vi "Func-엑셀 데이터를 그래프로 출력.vi"() -> ()   [LabVIEW 2015] (continued)
29.418\n25\t25\t29.423\n25\t25\t29.426\n25\t25\t29.429\n25\t25\t29.431\n25\t25\t29.437\n25\t25\t29.438\n25\t25\t29.442\n25\t25\t29.448\n25\t25\t29.456\n25\t25\t29.462\n25\t25\t29.462\n25\t25\t29.467\n25\t25\t29.473\n25\t25\t29.48\n25\t25\t29.483\n25\t25\t29.488\n25\t25\t29.499\n25\t25\t29.505\n25\t25\t29.508\n25\t25\t29.516\n25\t25\t29.517\n25\t25\t29.518\n25\t25\t29.519\n25\t25\t29.522\n25\t25\t29.527\n25\t25\t29.529\n25\t25\t29.536\n25\t25\t29.544\n25\t25\t29.548\n25\t25\t29.554\n25\t25\t29.559\n25\t25\t29.562\n25\t25\t29.565\n25\t25\t29.569\n25\t25\t29.576\n25\t25\t29.58\n25\t25\t29.585\n25\t25\t29.589\n25\t25\t29.595\n25\t25\t29.598\n25\t25\t29.604\n25\t25\t29.607\n25\t25\t29.609\n25\t25\t29.611\n25\t25\t29.611\n25\t25\t29.617\n25\t25\t29.616\n25\t25\t29.621\n25\t25\t29.626\n25\t25\t29.632\n25\t25\t29.64\n25\t25\t29.644\n25\t25\t29.651\n25\t25\t29.655\n25\t25\t29.661\n25\t25\t29.664\n25\t25\t29.663\n25\t25\t29.668\n25\t25\t29.669\n25\t25\t29.671\n25\t25\t29.68\n25\t25\t29.681\n25\t25\t29.686\n25\t25\t29.693\n25\t25\t29.7\n25\t25\t29.705\n25\t25\t29.707\n25\t25\t29.713\n25\t25\t29.716\n25\t25\t29.72\n25\t25\t29.721\n25\t25\t29.728\n25\t25\t29.73\n25\t25\t29.73\n25\t25\t29.734\n25\t25\t29.736\n25\t25\t29.74\n25\t25\t29.743\n25\t25\t29.75\n25\t25\t29.755\n25\t25\t29.756\n25\t25\t29.76\n25\t25\t29.762\n25\t25\t29.768\n25\t25\t29.77\n25\t25\t29.772\n25\t25\t29.783\n25\t25\t29.79\n25\t25\t29.794\n25\t25\t29.8\n25\t25\t29.803\n25\t25\t29.809\n25\t25\t29.811\n25\t25\t29.811\n25\t25\t29.815\n25\t25\t29.818\n25\t25\t29.825\n25\t25\t29.829\n25\t25\t29.836\n25\t25\t29.842\n25\t25\t29.846\n25\t25\t29.851\n25\t25\t29.854\n25\t25\t29.855\n25\t25\t29.859\n25\t25\t29.861\n25\t25\t29.866\n25\t25\t29.871\n25\t25\t29.871\n25\t25\t29.877\n25\t25\t29.881\n25\t25\t29.884\n25\t25\t29.885\n25\t25\t29.889\n25\t25\t29.894\n25\t25\t29.899\n25\t25\t29.902\n25\t25\t29.906\n25\t25\t29.913\n25\t25\t29.916\n25\t25\t29.92\n25\t25\t29.92\n25\t25\t29.923\n25\t25\t29.926\n25\t25\t29.927\n25\t25\t29.932\n25\t25\t29.935\n25\t25\t29.942\n25\t25\t29.949\n25\t25\t29.954\n25\t25\t29.964\n25\t25\t29.962\n25\t25\t29.966\n25\t25\t29.97\n25\t25\t29.97\n25\t25\t29.972\n25\t25\t29.972\n25\t25\t29.977\n25\t25\t29.982\n25\t25\t29.986\n25\t25\t29.99\n25\t25\t29.996\n25\t25\t30.006\n25\t25\t30.008\n25\t25\t30.011\n25\t25\t30.013\n25\t25\t30.017\n25\t25\t30.014\n25\t25\t30.016\n25\t25\t30.017\n25\t25\t30.025\n25\t25\t30.032\n25\t25\t30.036\n25\t25\t30.043\n25\t25\t30.047\n25\t25\t30.054\n25\t25\t30.055\n25\t25\t30.056\n25\t25\t30.061\n25\t25\t30.066\n25\t25\t30.069\n25\t25\t30.07\n25\t25\t30.075\n25\t25\t30.079\n25\t25\t30.083\n25\t25\t30.087\n25\t25\t30.093\n25\t25\t30.096\n25\t25\t30.098\n25\t25\t30.1\n25\t25\t30.098\n25\t25\t30.101\n25\t25\t30.104\n25\t25\t30.11\n25\t25\t30.114\n25\t25\t30.115\n25\t25\t30.119\n25\t25\t30.125\n25\t25\t30.127\n25\t25\t30.129\n25\t25\t30.138\n25\t25\t30.145\n25\t25\t30.15\n25\t25\t30.153\n25\t25\t30.154\n25\t25\t30.158\n25\t25\t30.154\n25\t25\t30.16\n25\t25\t30.165\n25\t25\t30.168\n25\t25\t30.174\n25\t25\t30.18\n25\t25\t30.186\n25\t25\t30.186\n25\t25\t30.19\n25\t25\t30.194\n25\t25\t30.197\n25\t25\t30.2\n25\t25\t30.203\n25\t25\t30.207\n25\t25\t30.212\n25\t25\t30.214\n25\t25\t30.218\n25\t25\t30.225\n25\t25\t30.226\n25\t25\t30.229\n25\t25\t30.229\n25\t25\t30.233\n25\t25\t30.234\n25\t25\t30.236\n25\t25\t30.243\n25\t25\t30.245\n25\t25\t30.249\n25\t25\t30.251\n25\t25\t30.253\n25\t25\t30.257\n25\t25\t30.257\n25\t25\t30.259\n25\t25\t30.264\n25\t25\t30.267\n25\t25\t30.272\n25\t25\t30.276\n25\t25\t30.282\n25\t25\t30.29\n25\t25\t30.293\n25\t25\t30.297\n25\t25\t30.302\n25\t25\t30.301\n25\t25\t30.301\n25\t25\t30.305\n25\t25\t30.306\n25\t25\t30.307\n25\t25\t30.312\n25\t25\t30.32\n25\t25\t30.326\n25\t25\t30.333\n25\t25\t30.338\n25\t25\t30.342\n25\t25\t30.343\n25\t25\t30.341\n25\t25\t30.346\n25\t25\t30.348\n25\t25\t30.346\n25\t25\t30.347\n25\t25\t30.352\n25\t25\t30.359\n25\t25\t30.356\n25\t25\t30.36\n25\t25\t30.366\n25\t25\t30.37\n25\t25\t30.372\n25\t25\t30.371\n25\t25\t30.38\n25\t25\t30.378\n25\t25\t30.381\n25\t25\t30.389\n25\t25\t30.391\n25\t25\t30.395\n25\t25\t30.399\n25\t25\t30.407\n25\t25\t30.41\n25\t25\t30.412\n25\t25\t30.415\n25\t25\t30.418\n25\t25\t30.422\n25\t25\t30.425\n25\t25\t30.431\n25\t25\t30.43\n25\t25\t30.434\n25\t25\t30.438\n25\t25\t30.443\n25\t25\t30.443\n25\t25\t30.442\n25\t25\t30.45\n25\t25\t30.452\n25\t25\t30.455\n25\t25\t30.459\n25\t25\t30.465\n25\t25\t30.468\n25\t25\t30.47\n25\t25\t30.471\n25\t25\t30.475\n25\t25\t30.477\n25\t25\t30.478\n25\t25\t30.484\n25\t25\t30.491\n25\t25\t30.495\n25\t25\t30.495\n25\t25\t30.5\n25\t25\t30.5\n25\t25\t30.503\n25\t25\t30.504\n25\t25\t30.51\n25\t25\t30.514\n25\t25\t30.516\n25\t25\t30.524\n25\t25\t30.529\n25\t25\t30.531\n25\t25\t30.533\n25\t25\t30.537\n25\t25\t30.539\n25\t25\t30.54\n25\t25\t30.54\n25\t25\t30.546\n25\t25\t30.547\n25\t25\t30.55\n25\t25\t30.553\n25\t25\t30.555\n25\t25\t30.558\n25\t25\t30.558\n25\t25\t30.562\n25\t25\t30.564\n25\t25\t30.567\n25\t25\t30.571\n25\t25\t30.573\n25\t25\t30.58\n25\t25\t30.579\n25\t25\t30.582\n25\t25\t30.583\n25\t25\t30.587\n25\t25\t30.591\n25\t25\t30.588\n25\t25\t30.589\n25\t25\t30.592\n25\t25\t30.597\n25\t25\t30.598\n25\t25\t30.603\n25\t25\t30.608\n25\t25\t30.616\n25\t25\t30.625\n25\t25\t30.629\n25\t25\t30.63\n25\t25\t30.635\n25\t25\t30.638\n25\t25\t30.637\n25\t25\t30.637\n25\t25\t30.64\n25\t25\t30.645\n25\t25\t30.647\n25\t25\t30.651\n25\t25\t30.659\n25\t25\t30.663\n25\t25\t30.665\n25\t25\t30.668\n25\t25\t30.668\n25\t25\t30.67\n25\t25\t30.672\n25\t25\t30.673\n25\t25\t30.677\n25\t25\t30.681\n25\t25\t30.686\n25\t25\t30.688\n25\t25\t30.691\n25\t25\t30.696\n25\t25\t30.697\n25\t25\t30.702\n25\t25\t30.705\n25\t25\t30.704\n25\t25\t30.707\n25\t25\t30.707\n25\t25\t30.711\n25\t25\t30.715\n25\t25\t30.72\n25\t25\t30.723\n25\t25\t30.725\n25\t25\t30.73\n25\t25\t30.729\n25\t25\t30.73\n25\t25\t30.729\n25\t25\t30.739\n25\t25\t30.741\n25\t25\t30.739\n25\t25\t30.745\n25\t25\t30.748\n25\t25\t30.749\n25\t25\t30.749\n25\t25\t30.75\n25\t25\t30.756\n25\t25\t30.761\n25\t25\t30.763\n25\t25\t30.77\n25\t25\t30.771\n25\t25\t30.777\n25\t25\t30.779\n25\t25\t30.781\n25\t25\t30.782\n25\t25\t30.777\n25\t25\t30.783\n25\t25\t30.785\n25\t25\t30.784\n25\t25\t30.786\n25\t25\t30.79\n25\t25\t30.796\n25\t25\t30.799\n25\t25\t30.8\n25\t25\t30.802\n25\t25\t30.806\n25\t25\t30.806\n25\t25\t30.807\n25\t25\t30.809\n25\t25\t30.814\n25\t25\t30.818\n25\t25\t30.821\n25\t25\t30.827\n25\t25\t30.831\n25\t25\t30.837\n25\t25\t30.837\n25\t25\t30.841\n25\t25\t30.845\n25\t25\t30.846\n25\t25\t30.846\n25\t25\t30.848\n25\t25\t30.85\n25\t25\t30.854\n25\t25\t30.855\n25\t25\t30.856\n25\t25\t30.865\n25\t25\t30.864\n25\t25\t30.869\n25\t25\t30.87\n25\t25\t30.875\n25\t25\t30.88\n25\t25\t30.878\n25\t25\t30.88\n25\t25\t30.885\n25\t25\t30.888\n25\t25\t30.889\n25\t25\t30.892\n25\t25\t30.895\n25\t25\t30.9\n25\t25\t30.897\n25\t25\t30.901\n25\t25\t30.903\n25\t25\t30.901\n25\t25\t30.905\n25\t25\t30.908\n25\t25\t30.913\n25\t25\t30.914\n25\t25\t30.916\n25\t25\t30.921\n25\t25\t30.923\n25\t25\t30.922\n25\t25\t30.926\n25\t25\t30.93\n25\t25\t30.931\n25\t25\t30.937\n25\t25\t30.939\n25\t25\t30.947\n25\t25\t30.953\n25\t25\t30.956\n25\t25\t30.959\n25\t25\t30.961\n25\t25\t30.965\n25\t25\t30.965\n25\t25\t30.966\n25\t25\t30.968\n25\t25\t30.972\n25\t25\t30.975\n25\t25\t30.974\n25\t25\t30.975\n25\t25\t30.978\n25\t25\t30.981\n25\t25\t30.981\n25\t25\t30.98\n25\t25\t30.985\n25\t25\t30.988\n25\t25\t30.997\n25\t25\t30.998\n25\t25\t31.003\n25\t25\t31.009\n25\t25\t31.011\n25\t25\t31.013\n25\t25\t31.01\n25\t25\t31.012\n25\t25\t31.011\n25\t25\t31.014\n25\t25\t31.014\n25\t25\t31.019\n25\t25\t31.021\n25\t25\t31.026\n25\t25\t31.029\n25\t25\t31.029\n25\t25\t31.033\n25\t25\t31.03\n25\t25\t31.037\n25\t25\t31.038\n25\t25\t31.043\n25\t25\t31.048\n25\t25\t31.05\n25\t25\t31.054\n25\t25\t31.055\n25\t25\t31.054\n25\t25\t31.055\n25\t25\t31.05\n25\t25\t31.051\n25\t25\t31.054\n25\t25\t31.053\n25\t25\t31.059\n25\t25\t31.061\n25\t25\t31.066\n25\t25\t31.07\n25\t25\t31.073\n25\t25\t31.078\n25\t25\t31.08\n25\t25\t31.081\n25\t25\t31.083\n25\t25\t31.086\n25\t25\t31.084\n25\t25\t31.086\n25\t25\t31.084\n25\t25\t31.089\n25\t25\t31.093\n25\t25\t31.096\n25\t25\t31.103\n25\t25\t31.104\n25\t25\t31.108\n25\t25\t31.114\n25\t25\t31.115\n25\t25\t31.12\n25\t25\t31.12\n25\t25\t31.123\n25\t25\t31.126\n25\t25\t31.125\n25\t25\t31.129\n25\t25\t31.132\n25\t25\t31.134\n25\t25\t31.133\n25\t25\t31.139\n25\t25\t31.141\n25\t25\t31.144\n25\t25\t31.145\n25\t25\t31.146\n25\t25\t31.149\n25\t25\t31.149\n25\t25\t31.15\n25\t25\t31.148\n25\t25\t31.148\n25\t25\t31.148\n25\t25\t31.15\n25\t25\t31.154\n25\t25\t31.154\n25\t25\t31.159\n25\t25\t31.164\n25\t25\t31.168\n25\t25\t31.168\n25\t25\t31.171\n25\t25\t31.175\n25\t25\t31.179\n25\t25\t31.181\n25\t25\t31.185\n25\t25\t31.188\n25\t25\t31.19\n25\t25\t31.19\n25\t25\t31.186\n25\t25\t31.19\n25\t25\t31.192\n25\t25\t31.195\n25\t25\t31.196\n25\t25\t31.204\n25\t25\t31.208\n25\t25\t31.21\n25\t25\t31.213\n25\t25\t31.218\n25\t25\t31.219\n25\t25\t31.219\n25\t25\t31.225\n25\t25\t31.227\n25\t25\t31.228\n25\t25\t31.232\n25\t25\t31.237\n25\t25\t31.237\n25\t25\t31.234\n25\t25\t31.238\n25\t25\t31.241\n25\t25\t31.242\n25\t25\t31.241\n25\t25\t31.245\n25\t25\t31.252\n25\t25\t31.254\n25\t25\t31.255\n25\t25\t31.253\n25\t25\t31.256\n25\t25\t31.259\n25\t25\t31.26\n25\t25\t31.261\n25\t25\t31.263\n25\t25\t31.265\n25\t25\t31.265\n25\t25\t31.265\n25\t25\t31.266\n25\t25\t31.27\n25\t25\t31.274\n25\t25\t31.279\n25\t25\t31.284\n25\t25\t31.288\n25\t25\t31.29\n25\t25\t31.289\n25\t25\t31.288\n25\t25\t31.289\n25\t25\t31.289\n25\t25\t31.293\n25\t25\t31.297\n25\t25\t31.3\n25\t25\t31.303\n25\t25\t31.306\n25\t25\t31.309\n25\t25\t31.311\n25\t25\t31.312\n25\t25\t31.313\n25\t25\t31.319\n25\t25\t31.321\n25\t25\t31.32\n25\t25\t31.321\n25\t25\t31.323\n25\t25\t31.326\n25\t25\t31.328\n25\t25\t31.33\n25\t25\t31.334\n25\t25\t31.336\n25\t25\t31.335\n25\t25\t31.335\n25\t25\t31.334\n25\t25\t31.333\n25\t25\t31.338\n25\t25\t31.339\n25\t25\t31.346\n25\t25\t31.355\n25\t25\t31.359\n25\t25\t31.366\n25\t25\t31.37\n25\t25\t31.371\n25\t25\t31.37\n25\t25\t31.366\n25\t25\t31.368\n25\t25\t31.366\n25\t25\t31.365\n25\t25\t31.366\n25\t25\t31.368\n25\t25\t31.374\n25\t25\t31.378\n25\t25\t31.38\n25\t25\t31.383\n25\t25\t31.389\n25\t25\t31.396\n25\t25\t31.394\n25\t25\t31.393\n25\t25\t31.398\n25\t25\t31.398\n25\t25\t31.397\n25\t25\t31.391\n25\t25\t31.391\n25\t25\t31.393\n25\t25\t31.392\n25\t25\t31.396\n25\t25\t31.396\n25\t25\t31.405\n25\t25\t31.409\n25\t25\t31.412\n25\t25\t31.418\n25\t25\t31.42\n25\t25\t31.418\n25\t25\t31.422\n25\t25\t31.423\n25\t25\t31.423\n25\t25\t31.422\n25\t25\t31.423\n25\t25\t31.428\n25\t25\t31.426\n25\t25\t31.429\n25\t25\t31.429\n25\t25\t31.432\n25\t25\t31.432\n25\t25\t31.431\n25\t25\t31.436\n25\t25\t31.437\n25\t25\t31.441\n25\t25\t31.446\n25\t25\t31.449\n25\t25\t31.455\n25\t25\t31.458\n25\t25\t31.462\n25\t25\t31.462\n25\t25\t31.458\n25\t25\t31.457\n25\t25\t31.46\n25\t25\t31.462\n25\t25\t31.464\n25\t25\t31.467\n25\t25\t31.471\n25\t25\t31.477\n25\t25\t31.475\n25\t25\t31.474\n25\t25\t31.473\n25\t25\t31.477\n25\t25\t31.479\n25\t25\t31.478\n25\t25\t31.482\n25\t25\t31.486\n25\t25\t31.491\n25\t25\t31.496\n25\t25\t31.496\n25\t25\t31.5\n25\t25\t31.501\n25\t25\t31.503\n25\t25\t31.5\n25\t25\t31.499\n25\t25\t31.503\n25\t25\t31.504\n25\t25\t31.511\n25\t25\t31.512\n25\t25\t31.515\n25\t25\t31.517\n25\t25\t31.515\n25\t25\t31.516\n25\t25\t31.52\n25\t25\t31.517\n25\t25\t31.518\n25\t25\t31.52\n25\t25\t31.526\n25\t25\t31.525\n25\t25\t31.522\n25\t25\t31.528\n25\t25\t31.531\n25\t25\t31.533\n25\t25\t31.531\n25\t25\t31.532\n25\t25\t31.536\n25\t25\t31.534\n25\t25\t31.536\n25\t25\t31.534\n25\t25\t31.538\n25\t25\t31.546\n25\t25\t31.548\n25\t25\t31.547\n25\t25\t31.554\n25\t25\t31.561\n25\t25\t31.561\n25\t25\t31.565\n25\t25\t31.568\n25\t25\t31.573\n25\t25\t31.575\n25\t25\t31.575\n25\t25\t31.577\n25\t25\t31.573\n25\t25\t31.572\n25\t25\t31.575\n25\t25\t31.577\n25\t25\t31.577\n25\t25\t31.578\n25\t25\t31.583\n25\t25\t31.585\n25\t25\t31.587\n25\t25\t31.587\n25\t25\t31.592\n25\t25\t31.596\n25\t25\t31.596\n25\t25\t31.601\n25\t25\t31.604\n25\t25\t31.605\n25\t25\t31.608\n25\t25\t31.61\n25\t25\t31.611\n25\t25\t31.607\n25\t25\t31.607\n25\t25\t31.607\n25\t25\t31.602\n25\t25\t31.604\n25\t25\t31.607\n25\t25\t31.612\n25\t25\t31.612\n25\t25\t31.618\n25\t25\t31.621\n25\t25\t31.621\n25\t25\t31.62\n25\t25\t31.62\n25\t25\t31.625\n25\t25\t31.626\n25\t25\t31.626\n25\t25\t31.631\n25\t25\t31.637\n25\t25\t31.639\n25\t25\t31.641\n25\t25\t31.641\n25\t25\t31.65\n25\t25\t31.649\n25\t25\t31.65\n25\t25\t31.649\n25\t25\t31.652\n25\t25\t31.65\n25\t25\t31.651\n25\t25\t31.654\n25\t25\t31.656\n25\t25\t31.657\n25\t25\t31.655\n25\t25\t31.661\n25\t25\t31.659\n25\t25\t31.661\n25\t25\t31.661\n25\t25\t31.67\n25\t25\t31.674\n25\t25\t31.67\n25\t25\t31.671\n25\t25\t31.67\n25\t25\t31.668\n25\t25\t31.666\n25\t25\t31.664\n25\t25\t31.668\n25\t25\t31.671\n25\t25\t31.675\n25\t25\t31.68\n25\t25\t31.682\n25\t25\t31.686\n25\t25\t31.687\n25\t25\t31.69\n25\t25\t31.689\n25\t25\t31.691\n25\t25\t31.691\n25\t25\t31.693\n25\t25\t31.699\n25\t25\t31.698\n25\t25\t31.696\n25\t25\t31.698\n25\t25\t31.703\n25\t25\t31.702\n25\t25\t31.701\n25\t25\t31.704\n25\t25\t31.708\n25\t25\t31.707\n25\t25\t31.704\n25\t25\t31.71\n25\t25\t31.711\n25\t25\t31.714\n25\t25\t31.717\n25\t25\t31.72\n25\t25\t31.722\n25\t25\t31.721\n25\t25\t31.723\n25\t25\t31.723\n25\t25\t31.723\n25\t25\t31.727\n25\t25\t31.729\n25\t25\t31.733\n25\t25\t31.73\n25\t25\t31.735\n25\t25\t31.739\n25\t25\t31.736\n25\t25\t31.734\n25\t25\t31.735\n25\t25\t31.742\n25\t25\t31.743\n25\t25\t31.745\n25\t25\t31.75\n25\t25\t31.753\n25\t25\t31.755\n25\t25\t31.755\n25\t25\t31.757\n25\t25\t31.754\n25\t25\t31.755\n25\t25\t31.76\n25\t25\t31.763\n25\t25\t31.764\n25\t25\t31.764\n25\t25\t31.771\n25\t25\t31.77\n25\t25\t31.769\n25\t25\t31.771\n25\t25\t31.773\n25\t25\t31.774\n25\t25\t31.771\n25\t25\t31.777\n25\t25\t31.777\n25\t25\t31.779\n25\t25\t31.779\n25\t25\t31.781\n25\t25\t31.782\n25\t25\t31.779\n25\t25\t31.784\n25\t25\t31.787\n25\t25\t31.789\n25\t25\t31.791\n25\t25\t31.795\n25\t25\t31.798\n25\t25\t31.799\n25\t25\t31.801\n25\t25\t31.804\n25\t25\t31.804\n25\t25\t31.807\n25\t25\t31.811\n25\t25\t31.809\n25\t25\t31.81\n25\t25\t31.81\n25\t25\t31.811\n25\t25\t31.812\n25\t25\t31.813\n25\t25\t31.818\n25\t25\t31.821\n25\t25\t31.822\n25\t25\t31.823\n25\t25\t31.824\n25\t25\t31.823\n25\t25\t31.823\n25\t25\t31.821\n25\t25\t31.826\n25\t25\t31.826\n25\t25\t31.83\n25\t25\t31.832\n25\t25\t31.835\n25\t25\t31.838\n25\t25\t31.841\n25\t25\t31.847\n25\t25\t31.845\n25\t25\t31.845\n25\t25\t31.844\n25\t25\t31.844\n25\t25\t31.841\n25\t25\t31.841\n25\t25\t31.843\n25\t25\t31.844\n25\t25\t31.845\n25\t25\t31.848\n25\t25\t31.848\n25\t25\t31.849\n25\t25\t31.851\n25\t25\t31.854\n25\t25\t31.857\n25\t25\t31.855\n25\t25\t31.857\n25\t25\t31.861\n25\t25\t31.859\n25\t25\t31.862\n25\t25\t31.863\n25\t25\t31.864\n25\t25\t31.868\n25\t25\t31.869\n25\t25\t31.873\n25\t25\t31.874\n25\t25\t31.876\n25\t25\t31.878\n25\t25\t31.879\n25\t25\t31.882\n25\t25\t31.885\n25\t25\t31.883\n25\t25\t31.882\n25\t25\t31.882\n25\t25\t31.886\n25\t25\t31.885\n25\t25\t31.885\n25\t25\t31.888\n25\t25\t31.892\n25\t25\t31.895\n25\t25\t31.894\n25\t25\t31.895\n25\t25\t31.895\n25\t25\t31.898\n25\t25\t31.899\n25\t25\t31.901\n25\t25\t31.904\n25\t25\t31.906\n25\t25\t31.91\n25\t25\t31.911\n25\t25\t31.91\n25\t25\t31.909\n25\t25\t31.909\n25\t25\t31.909\n25\t25\t31.908\n25\t25\t31.911\n25\t25\t31.914\n25\t25\t31.917\n25\t25\t31.918\n25\t25\t31.921\n25\t25\t31.921\n25\t25\t31.922\n25\t25\t31.922\n25\t25\t31.925\n25\t25\t31.928\n25\t25\t31.927\n25\t25\t31.927\n25\t25\t31.928\n25\t25\t31.929\n25\t25\t31.927\n25\t25\t31.927\n25\t25\t31.93\n25\t25\t31.937\n25\t25\t31.936\n25\t25\t31.937\n25\t25\t31.942\n25\t25\t31.941\n25\t25\t31.941\n25\t25\t31.939\n25\t25\t31.942\n25\t25\t31.944\n25\t25\t31.947\n25\t25\t31.953\n25\t25\t31.955\n25\t25\t31.957\n25\t25\t31.96\n25\t25\t31.96\n25\t25\t31.961\n25\t25\t31.959\n25\t25\t31.958\n25\t25\t31.958\n25\t25\t31.957\n25\t25\t31.958\n25\t25\t31.959\n25\t25\t31.963\n25\t25\t31.966\n25\t25\t31.968\n25\t25\t31.968\n25\t25\t31.97\n25\t25\t31.973\n25\t25\t31.971\n25\t25\t31.976\n25\t25\t31.977\n25\t25\t31.979\n25\t25\t31.979\n25\t25\t31.978\n25\t25\t31.978\n25\t25\t31.976\n25\t25\t31.979\n25\t25\t31.981\n25\t25\t31.984\n25\t25\t31.987\n25\t25\t31.985\n25\t25\t31.989\n25\t25\t31.988\n25\t25\t31.992\n25\t25\t31.989\n25\t25\t31.989\n25\t25\t31.992\n25\t25\t31.991\n25\t25\t31.993\n25\t25\t31.993\n25\t25\t32\n25\t25\t32.006\n25\t25\t32.01\n25\t25\t32.011\n25\t25\t32.01\n25\t25\t32.012\n25\t25\t32.011\n25\t25\t32.008\n25\t25\t32.01\n25\t25\t32.011\n25\t25\t32.016\n25\t25\t32.016\n25\t25\t32.018\n25\t25\t32.021\n25\t25\t32.021\n25\t25\t32.022\n25\t25\t32.023\n25\t25\t32.024\n25\t25\t32.023\n25\t25\t32.021\n25\t25\t32.024\n25\t25\t32.023\n25\t25\t32.021\n25\t25\t32.022\n25\t25\t32.024\n25\t25\t32.027\n25\t25\t32.029\n25\t25\t32.03\n25\t25\t32.032\n25\t25\t32.036\n25\t25\t32.039\n25\t25\t32.038\n25\t25\t32.037\n25\t25\t32.042\n25\t25\t32.042\n25\t25\t32.043\n25\t25\t32.044\n25\t25\t32.047\n25\t25\t32.049\n25\t25\t32.048\n25\t25\t32.051\n25\t25\t32.051\n25\t25\t32.05\n25\t25\t32.048\n25\t25\t32.049\n25\t25\t32.048\n25\t25\t32.05\n25\t25\t32.056\n25\t25\t32.057\n25\t25\t32.061\n25\t25\t32.063\n25\t25\t32.066\n25\t25\t32.066\n25\t25\t32.064\n25\t25\t32.065\n25\t25\t32.066\n25\t25\t32.066\n25\t25\t32.067\n25\t25\t32.066\n25\t25\t32.069\n25\t25\t32.073\n25\t25\t32.071\n25\t25\t32.071\n25\t25\t32.072\n25\t25\t32.075\n25\t25\t32.074\n25\t25\t32.071\n25\t25\t32.078\n25\t25\t32.079\n25\t25\t32.078\n25\t25\t32.082\n25\t25\t32.083\n25\t25\t32.089\n25\t25\t32.086\n25\t25\t32.088\n25\t25\t32.091\n25\t25\t32.09\n25\t25\t32.09\n25\t25\t32.087\n25\t25\t32.087\n25\t25\t32.091\n25\t25\t32.095\n25\t25\t32.094\n25\t25\t32.095\n25\t25\t32.096\n25\t25\t32.099\n25\t25\t32.097\n25\t25\t32.093\n25\t25\t32.097\n25\t25\t32.104\n25\t25\t32.107\n25\t25\t32.108\n25\t25\t32.111\n25\t25\t32.116\n25\t25\t32.118\n25\t25\t32.114\n25\t25\t32.112\n25\t25\t32.112\n25\t25\t32.114\n25\t25\t32.114\n25\t25\t32.115\n25\t25\t32.116\n25\t25\t32.119\n25\t25\t32.121\n25\t25\t32.123\n25\t25\t32.123\n25\t25\t32.124\n25\t25\t32.127\n25\t25\t32.13\n25\t25\t32.133\n25\t25\t32.132\n25\t25\t32.13\n25\t25\t32.131\n25\t25\t32.13\n25\t25\t32.13\n25\t25\t32.13\n25\t25\t32.134\n25\t25\t32.137\n25\t25\t32.136\n25\t25\t32.137\n25\t25\t32.136\n25\t25\t32.137\n25\t25\t32.138\n25\t25\t32.139\n25\t25\t32.142\n25\t25\t32.144\n25\t25\t32.145\n25\t25\t32.146\n25\t25\t32.145\n25\t25\t32.146\n25\t25\t32.146\n25\t25\t32.148\n25\t25\t32.152\n25\t25\t32.152\n25\t25\t32.149\n25\t25\t32.154\n25\t25\t32.155\n25\t25\t32.153\n25\t25\t32.154\n25\t25\t32.154\n25\t25\t32.158\n25.083\t25.05\t32.775\n25.167\t25.12\t32.771\n25.25\t24.99\t32.783\n25.333\t24.95\t32.796\n25.417\t24.86\t32.794\n25.5\t24.74\t32.798\n25.583\t24.62\t32.788\n25.667\t24.49\t32.797\n25.75\t24.35\t32.799\n25.833\t24.24\t32.8\n25.917\t24.12\t32.8\n26\t24.03\t32.802\n26.083\t23.98\t32.808\n26.167\t23.94\t32.802\n26.25\t23.93\t32.809\n26.333\t23.95\t32.809\n26.417\t23.98\t32.812\n26.5\t24.03\t32.811\n26.583\t24.1\t32.814\n26.667\t24.19\t32.814\n26.75\t24.29\t32.811\n26.833\t24.41\t32.796\n26.917\t24.53\t32.803\n27\t24.65\t32.804\n27.083\t24.77\t32.811\n27.167\t24.89\t32.805\n27.25\t25.01\t32.805\n27.333\t25.13\t32.799\n27.417\t25.25\t32.799\n27.5\t25.35\t32.796\n27.583\t25.46\t32.798\n27.667\t25.58\t32.796\n27.75\t25.68\t32.797\n27.833\t25.77\t32.789\n27.917\t25.86\t32.791\n28\t25.94\t32.789\n28.083\t26.02\t32.793\n28.167\t26.09\t32.794\n28.25\t26.1\t32.792\n28.333\t26.16\t32.795\n28.417\t26.34\t32.804\n28.5\t26.6\t32.803\n28.583\t26.89\t32.804\n28.667\t27.19\t32.815\n28.75\t27.46\t32.819\n28.833\t27.69\t32.812\n28.917\t27.92\t32.829\n29\t28.11\t32.832\n29.083\t28.27\t32.843\n29.167\t28.4\t32.858\n29.25\t28.53\t32.868\n29.333\t28.64\t32.874\n29.417\t28.74\t32.884\n29.5\t28.82\t32.898\n29.583\t28.9\t32.914\n29.667\t28.98\t32.917\n29.75\t29.04\t32.941\n29.833\t29.11\t32.956\n29.917\t29.15\t32.976\n30\t29.21\t32.995\n30.083\t29.24\t33.002\n30.167\t29.28
